vi "Traverse-Settings-Global.vi"() -> ()   [LabVIEW 2017]
uses:
  Settings-Control.ctl
panel:
  in  "Settings":T1
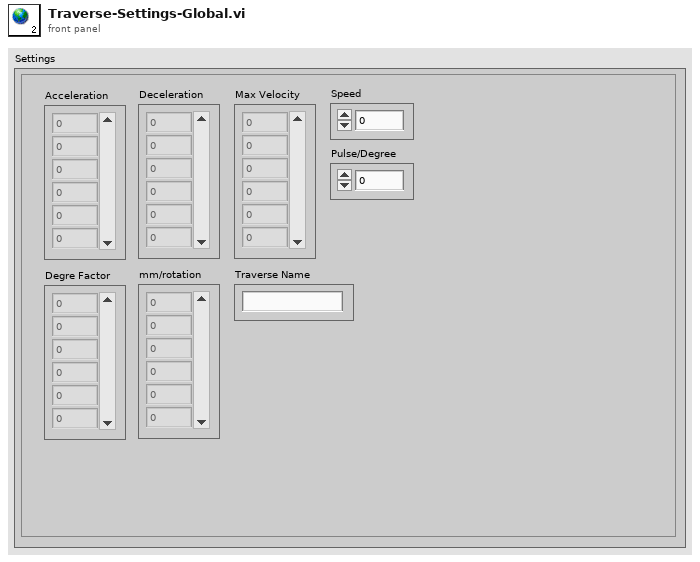
[diagram p1: front panel]
types:
  T1 = typedef "Settings-Control.ctl" = cluster{"Acceleration":dbl[], "Deceleration":dbl[], "Max Velocity":dbl[], "Speed":dbl, "Pulse/Degree":dbl, "Degre Factor":dbl[], "mm/rotation":dbl[], "Traverse Name":string}
diagram:
